vi "ExploreWeights.vi"() -> ()   [LabVIEW 2016]
uses:
  Controls/Type of Synapses.ctl
  <vilib>/Utility/xml.llb/Read From XML File(string).vi
  Cerebellum/Cerebellum.lvclass
  AER.lvclass
panel:
  out "Synaptic parameters":T2(array[cluster])
  out "PCBA idx":i32[](array[numeric])
  out "size(s)":i32
  out "GOGC idx":i32[](array[numeric])
  out "Pre IDs":i32[](array[numeric])
  out "No N":i32[](array[numeric])
  out "No Pre":i32[](array[numeric])
  out "Picture":picture
  out "Array":dbl[][](array[numeric])
  out "sum":i32
  in  "Right Hemis":path
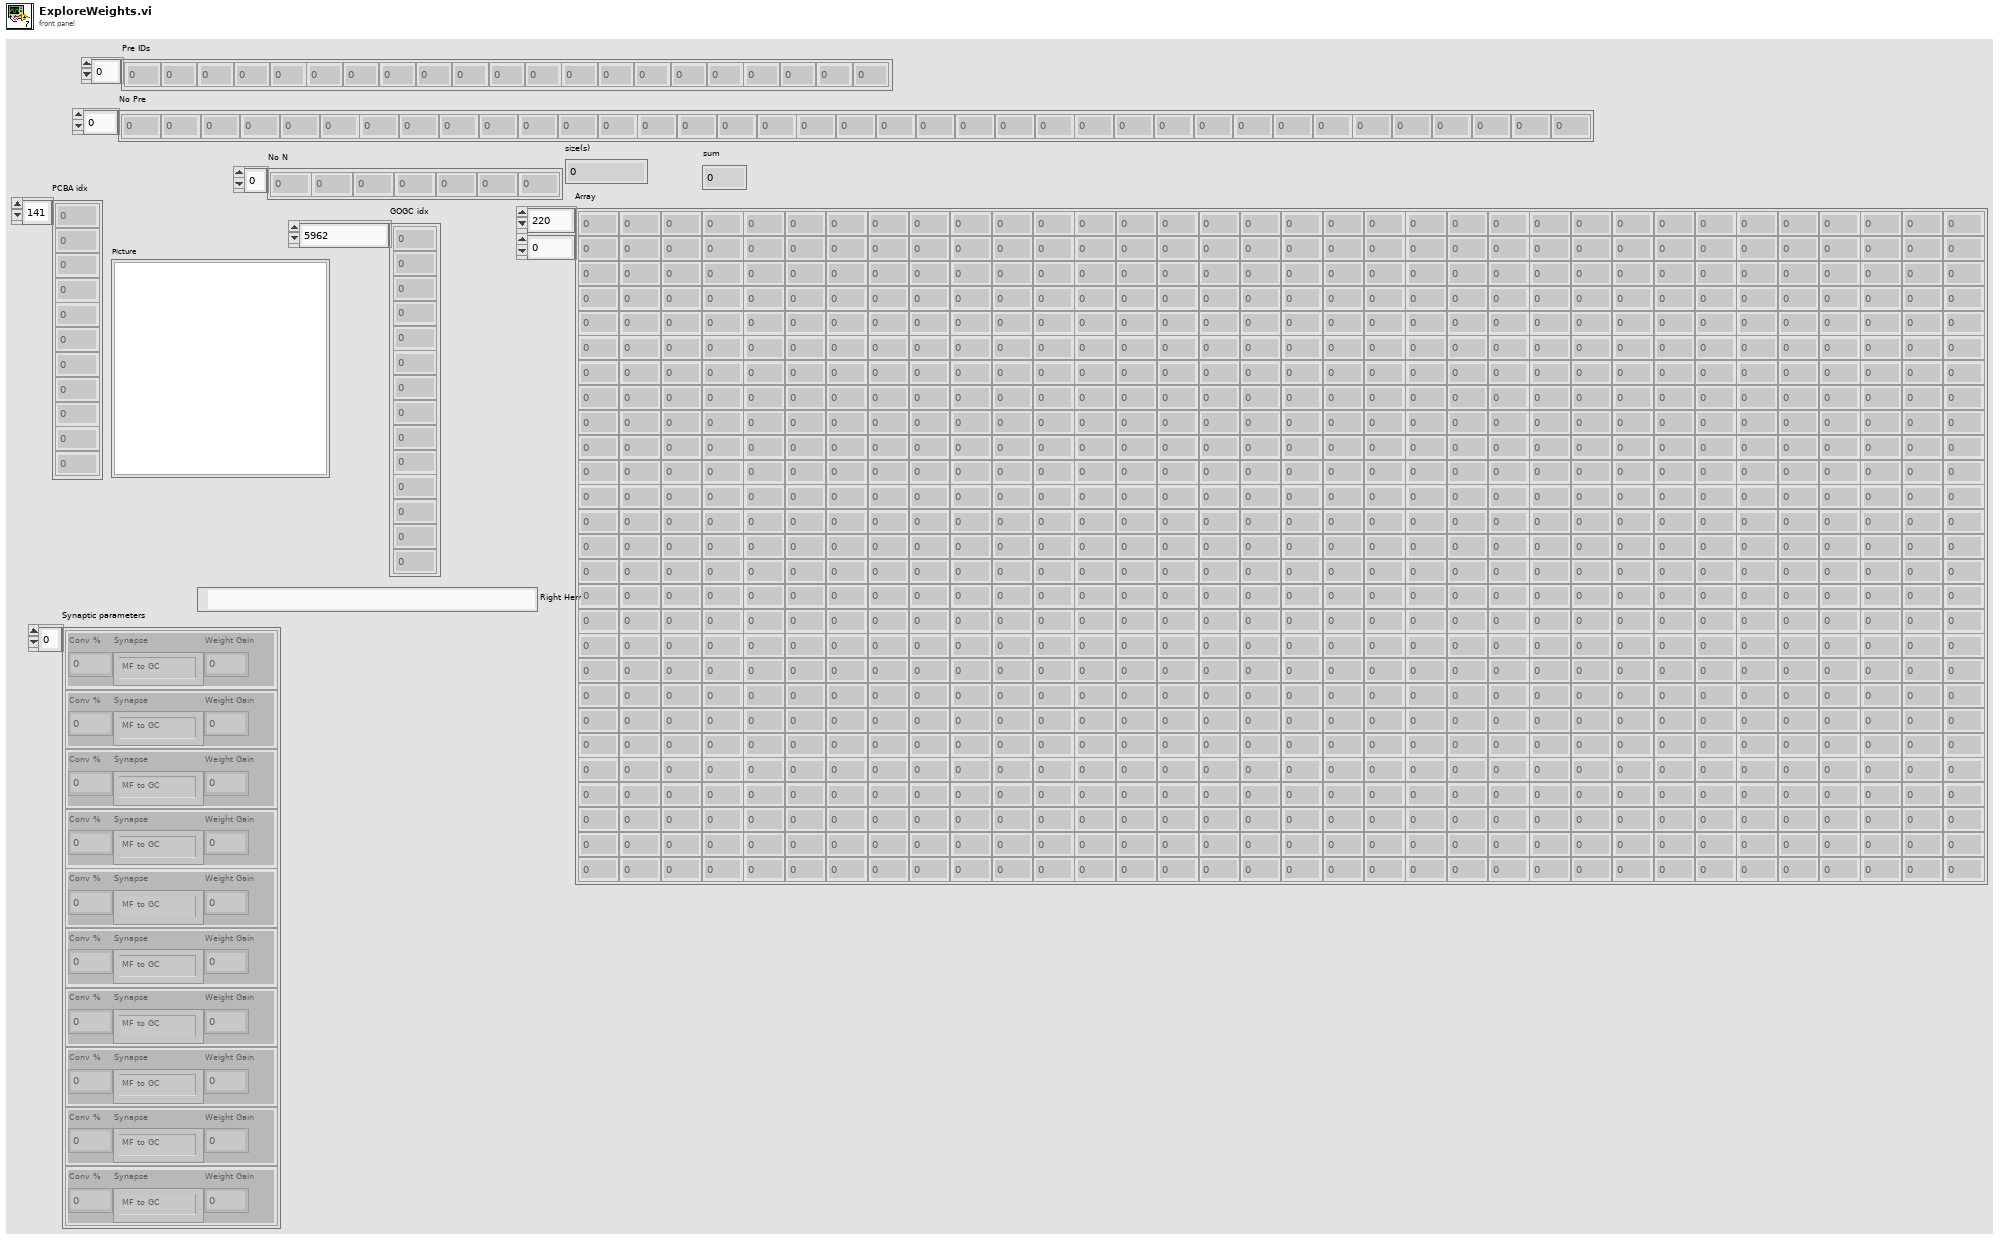
[diagram p1: front panel]
types:
  T1 = typedef "Type of Synapses.ctl" = enum16{"MF to GC", "GO to GC", "GC to GO", "MF to GO", "GC to PC", "GC to BA", "PC to BA", "BA to PC", "BA to GO"}
  T2 = cluster{"Conv %":dbl, "Synapse":T1, "Weight Gain":dbl}[]
  T3 = typedef "imagedata.ctl" = cluster{"image type":i32, "image depth":i32, "image":u8[], "mask":u8[], "colors":u32[], "Rectangle":cluster{"left":i16, "top":i16, "right":i16, "bottom":i16}}
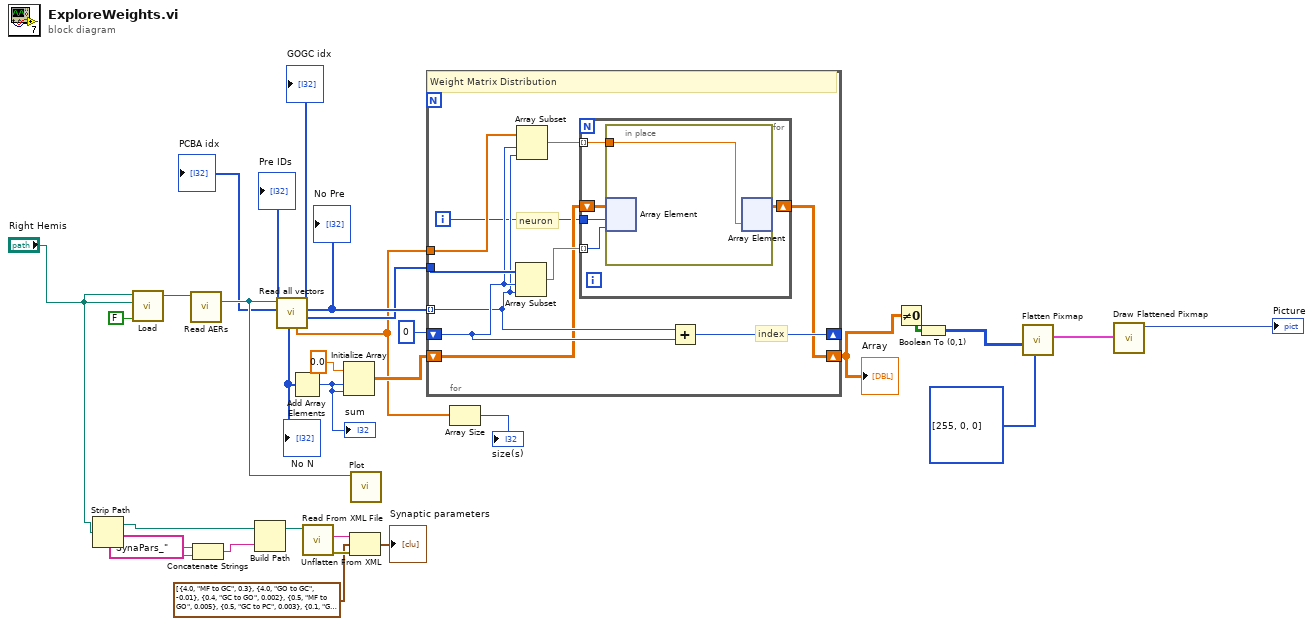
[diagram p0: block diagram]
diagram:
  n1 = Strip Path(path="Right Hemis") -> (stripped path=w9:path, name=w7:string)
  n2 = call "Load.vi"("Trained?"=FALSE, "Left Hem Path"="Right Hemis", "Right Hem Path"="Right Hemis") -> ("Cerebellum out"=w29:refnum<class "Cerebellum.lvclass">)  [unwired: 8 in]
  n3 = call-dynamic "Read AERs.vi"("Cerebellum in"=w29) -> ("AER Left"=w19:refnum<class "AER.lvclass">)  [unwired: 7 in, 3 out]
  n4 = Concatenate Strings("SynaPars_" ("string"), w7) -> (w6:string)
  n5 = Build Path(base path=w9, name or relative path=w6) -> (appended path=w8:path)
  n6 = call-dynamic "Read all vectors.vi"("AER in"=w19) -> ("Pre IDs"=w22:i32[], "No Pre"=w28:i32[], "W"=w13:dbl[], "No N"=w26:i32[], "GOGC idx"=→"GOGC idx":i32[], "PCBA idx"=→"PCBA idx":i32[])  [unwired: 1 in, 4 out]
  "No Pre" <- w28
  "No N" <- w26
  "Pre IDs" <- w22
  n7 = Add Array Elements(numeric array=w26) -> (sum=w25:i32)
  "sum" <- w25
  n8 = call-poly <vilib>:"Read From XML File.vi"("XML File Path"=w8) -> ("error out"=w4:errorcluster, "XML Elements"=w3:string)  [unwired: 8 in, 1 out]
  n9 = Initialize Array(0.0, w25, w25) -> (w23:dbl[][])
  n10 = Unflatten From XML(xml string=w3, type=T2 [{"Conv %"=4.0, "Synapse"=enum."MF to GC", "Weight Gain"=0.3}, {"Conv %"=4.0, "Synapse"=enum."GO to GC", "Weight Gain"=-0.01}, {"Conv %"=0.4, "Synapse"=enum."GC to GO", "Weight Gain"=0.002}, {"Conv %"=0.5, "Synapse"=enum."MF to GO", "Weight Gain"=0.005}, {"Conv %"=0.5, "Synapse"=enum."GC to PC", "Weight Gain"=0.003}, {"Conv %"=0.1, "Synapse"=enum."GC to BA", "Weight Gain"=0.01}, {"Conv %"=0.01, "Synapse"=enum."PC to BA", "Weight Gain"=-0.2}, {"Conv %"=0.4, "Synapse"=enum."BA to PC", "Weight Gain"=-0.01}, {"Conv %"=0.1, "Synapse"=enum."BA to GO", "Weight Gain"=-0.01}] ("Synapses and parameters"), error in (no error)=w4) -> (value=→"Synaptic parameters":T2)  [unwired: 1 out]
  n11 = call "Plot.vi"("AER in"=w19) -> ()  [unwired: 11 in]
  n12 = for {
    tunnel: w28 -> [w36] mode=indexing
    shift-right: [w40] -> _
    shift-left: 0 ("size(s)") -> [w37]
    shift-right: [w33] -> w18
    shift-left: w23 -> [w34]
    tunnel: w22 -> [w39]
    tunnel: w13 -> [w38]
    i -> [w31]
    # "neuron"
    # "index"
    # "Weight Matrix Distribution"
    n13 = Array Subset(array=w39, index=w37, length=w36) -> (w35:i32[])
    n14 = Array Subset(array=w38, index=w37, length=w36) -> (w32:dbl[])
    n15 = for {
      tunnel: w35 -> [w43] mode=indexing
      shift-right: [w44] -> w33
      shift-left: w34 -> [w45]
      tunnel: w32 -> [w42] mode=indexing
      tunnel: w31 -> [w41]
      n16 = in-place {
        in-place-border: w42 -> [w46]
        n17 = in-place-array #1(w45, w41, w43) -> ()  [unwired: 1 out]
        n18 = in-place-array #1(w46) -> (w44:dbl[][])  [unwired: 2 out]
      }
    }
    n19 = Add(x=w36, y=w37) -> (x+y=w40:i32)
  }
  "Array" <- w18
  n20 = Array Size(array=w13) -> (size(s)=→"size(s)":i32)
  n21 = Not Equal To 0?(x=w18) -> (x != 0?=w17:bool[][])
  n22 = Boolean To (0,1)(Boolean=w17) -> (0, 1=w16:i16[][])
  n23 = call <vilib>:"Flatten Pixmap.vi"("colors"=u32[] [255, 0, 0], "4-bit pixmap"=w16) -> ("image data"=w20:T3)  [unwired: 9 in]
  n24 = call <vilib>:"Draw Flattened Pixmap.vi"("image data"=w20) -> ("new picture"=→"Picture":picture)  [unwired: 8 in]
